vi "Disp Waveform with XY Graph.vi"() -> ()   [LabVIEW 2012]
uses:
  <vilib>/Waveform/WDTOps.llb/WDT Get Waveform Time Array DBL.vi
  <vilib>/Waveform/WDTOps.llb/WDT Waveform to XY Pairs DBL.vi
  <vilib>/measure/NI_MAPro.lvlib
panel:
  out "复数数组":cdb[](graph)
  out "XY数组捆绑":cluster{timestamp[], dbl[]}(graph)
  out "XY对簇数组":cluster{"x":timestamp, "y":dbl}[](graph)
  in  "tone amplitudes":dbl[](array[numeric])=[1.0, 1.0, 1.0, 1.0] caption="单频幅值"
  in  "tone frequencies":dbl[](array[numeric])=[100.0, 200.0, 300.0, 400.0] caption="单频频率"
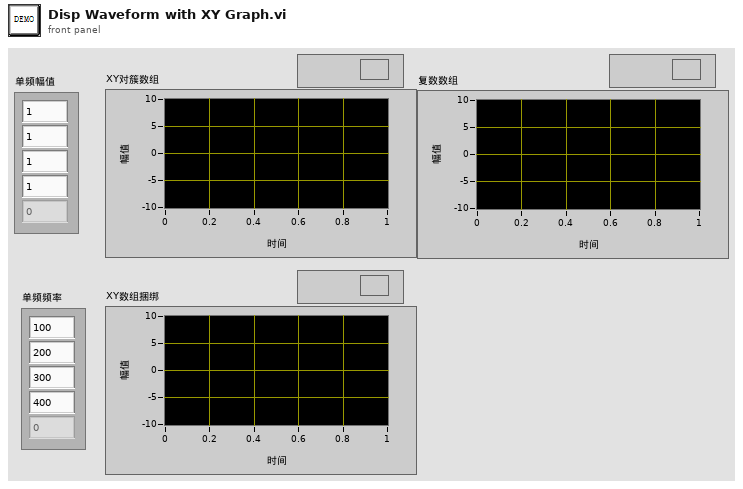
[diagram p1: front panel]
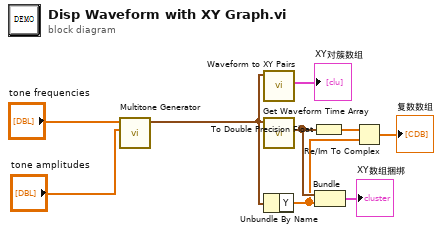
[diagram p0: block diagram]
diagram:
  n1 = call <vilib>:"Multitone Generator.vi"("tone amplitudes"="tone amplitudes", "tone frequencies"="tone frequencies") -> ("signal out"=w6:waveform(dbl))  [unwired: 6 in, 3 out]
  n2 = call-poly <vilib>:"Waveform to XY Pairs.vi"("waveform in"=w6) -> ("XY pairs"=→"XY对簇数组":cluster{"x":timestamp, "y":dbl}[])  [unwired: 8 in, 2 out]
  n3 = call-poly <vilib>:"Get Waveform Time Array.vi"("waveform in"=w6) -> ("X array"=w4:timestamp[])  [unwired: 9 in, 1 out]
  n4 = Unbundle By Name(w6) -> ("Y"=w2:dbl[])
  n5 = To Double Precision Float(number=w4) -> (double precision float=w3:dbl[])
  n6 = Bundle("X array"=w4, "Y"=w2) -> (→"XY数组捆绑":cluster{"X array":timestamp[], "Y":dbl[]})  [unwired: 1 in]
  n7 = Re/Im To Complex(1:w2, 2:w3) -> (0:→"复数数组":cdb[])
